vi "setFmat.vi"(7 "tolerance":dbl=1e-15 format="%.2e", 8 "error in (no error)":errorcluster, 9 "dofIdx":i16[](array[numeric]), 10 "Q Matrix":dbl[][](array[numeric]), 11 "OptCtrl in":refnum<class "OptCtrl.lvclass">) -> (0 "error out":errorcluster, 3 "OptCtrl out":refnum<class "OptCtrl.lvclass">)   [LabVIEW 2016, in "OptCtrl.lvclass"]
doc: "Set the F matrix. F = pinv(A.T * C.T * C * A + rho * H)."
uses:
  OptCtrl.lvclass
  OptCtrl.lvclass/OptCtrl.ctl
  <vilib>/Analysis/_algsub.llb/Real PseudoInverse Matrix.vi
  Utility/getSubArray2D.vi
  <vilib>/Analysis/Matrix/Numeric/Conversions/Matrix To Array - RM.vi
  <vilib>/Analysis/NI_AALPro.lvlib
  <vilib>/Analysis/Matrix/NI_Matrix.lvlib
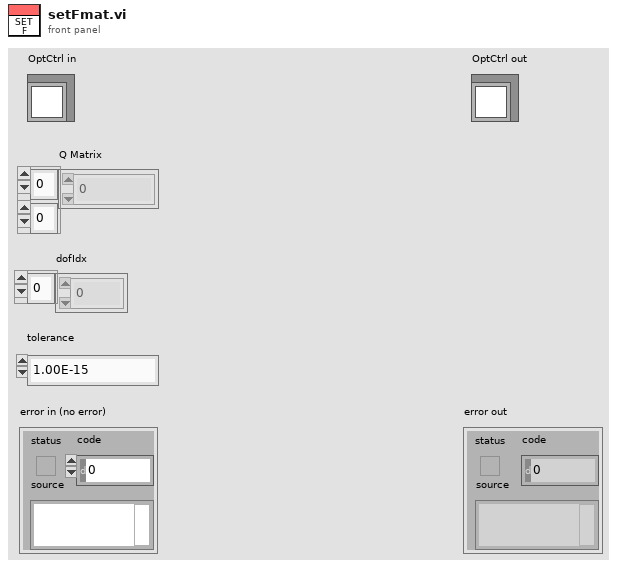
[diagram p1: front panel]
types:
  T1 = typedef "NI_Matrix.lvlib/RealMatrix.ctl" = dbl[][]
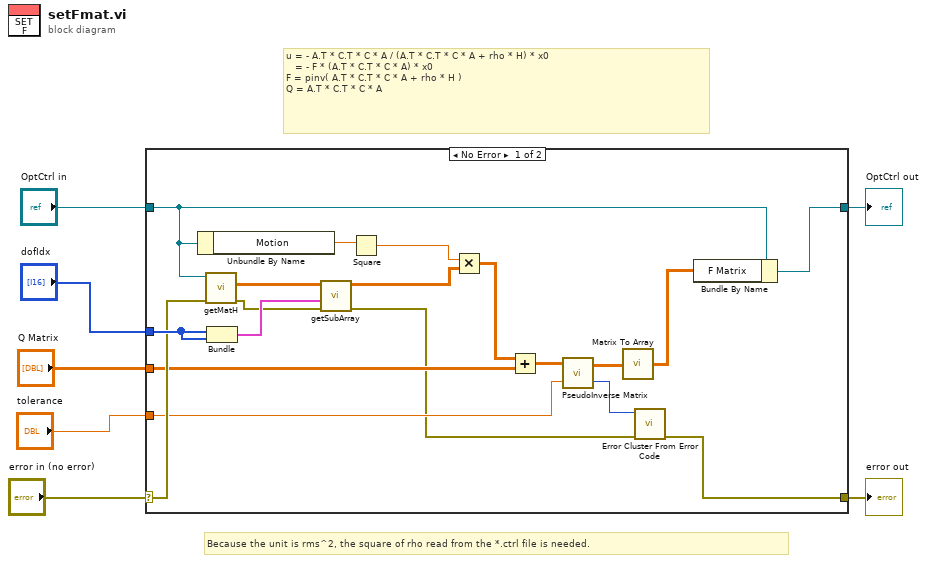
[diagram p0: block diagram]
diagram:
  # "Because the unit is rms^2, the square of rho read from the *.ctrl file is needed."
  # "u = - A.T * C.T * C * A / (A.T * C.T * C * A + rho * H) * x0\n   = - F * (A.T * C.T * C * A) * x0\nF = pinv( A.T * C.T * C * A + rho * H )\nQ = A.T * C.T * C * A"
  n1 = case shown="No Error" "error in (no error)" {
    selector: "error in (no error)" -> [w22 w28]
    tunnel: [w12 w28] -> w6
    tunnel: [w8 w27] -> w4
    tunnel: "OptCtrl in" -> [w10 w27]
    tunnel: "dofIdx" -> [w24 _]
    tunnel: "Q Matrix" -> [w17 _]
    tunnel: "tolerance" -> [w15 _]
    frame No Error {
      n2 = Unbundle By Name(w10) -> ("Motion"=w26:dbl)
      n3 = call "getMatH.vi"("error in (no error)"=w22, "OptCtrl in"=w10) -> ("error out"=w21:errorcluster, "Matrix H"=w25:dbl[][])  [unwired: 7 in, 1 out]
      n4 = Bundle("dofIdx"=w24, "dofIdx"=w24) -> (w23:cluster{"dofIdx":i16[], "dofIdx":i16[]})  [unwired: 1 in]
      n5 = call-poly "getSubArray.vi"("error in (no error)"=w21, "Index Array Cluster"=w23, "2D Array"=w25) -> ("error out"=w13:errorcluster, "Sub-Array"=w19:dbl[][])  [unwired: 7 in]
      n6 = Square(x=w26) -> (x^2=w20:dbl)
      n7 = Multiply(x=w20, y=w19) -> (x*y=w18:dbl[][])
      n8 = Add(x=w18, y=w17) -> (x+y=w16:dbl[][])
      n9 = call-poly <vilib>:"PseudoInverse Matrix.vi"("tolerance"=w15, "Input Matrix"=w16) -> ("error"=w14:i32, "PseudoInverse Matrix"=w11:T1)
      n10 = call-poly <vilib>:"Matrix To Array.vi"("Real Matrix"=w11) -> ("Real 2D Array"=w9:dbl[][])
      n11 = call <vilib>:"Error Cluster From Error Code.vi"("error in (no error)"=w13, "error code (0)"=w14) -> ("error out"=w12:errorcluster)  [unwired: 7 in]
      n12 = Bundle By Name(cluster=w10, "F Matrix"=w9) -> (w8:refnum<class "OptCtrl.lvclass">)
    }
    frame Error {
    }
  }
  "error out" <- w6
  "OptCtrl out" <- w4
